vi "c ctre phoenixpro Request Control Position Voltage.vi"(0 "canbus":string, 1 "Position":dbl, 2 "FeedForward":dbl, 5 "ecuEncoding":u32, 7 "updateTime":dbl, 9 "cancelOtherRequests":bool, 11 "error in (no error)":errorcluster, 12 "EnableFOC":bool, 13 "Slot":i32) -> (4 "function return":i32, 15 "error out":errorcluster)   [LabVIEW 2020, in "CTRE_PhoenixTools.lvlib"]
doc: "CTREXPORT int c_ctre_phoenixpro_RequestControlPositionVoltage(const char *canbus, uint32_t ecuEncoding, double updateTime, bool cancelOtherRequests, double Position, bool EnableFOC, double FeedForward, int Slot);"
uses:
  <userlib>/CTRE_PhoenixTools/CTRE_PhoenixTools.lvlib
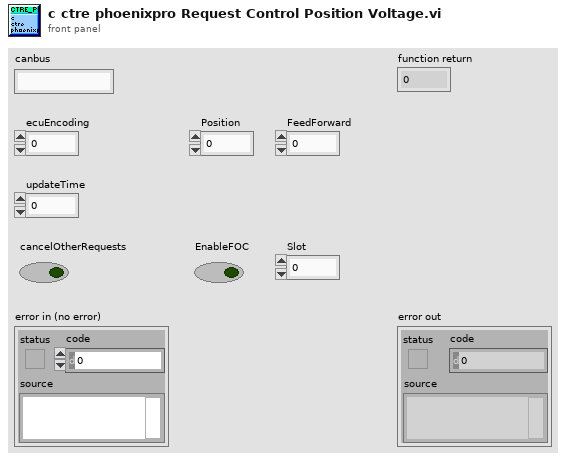
[diagram p1: front panel]
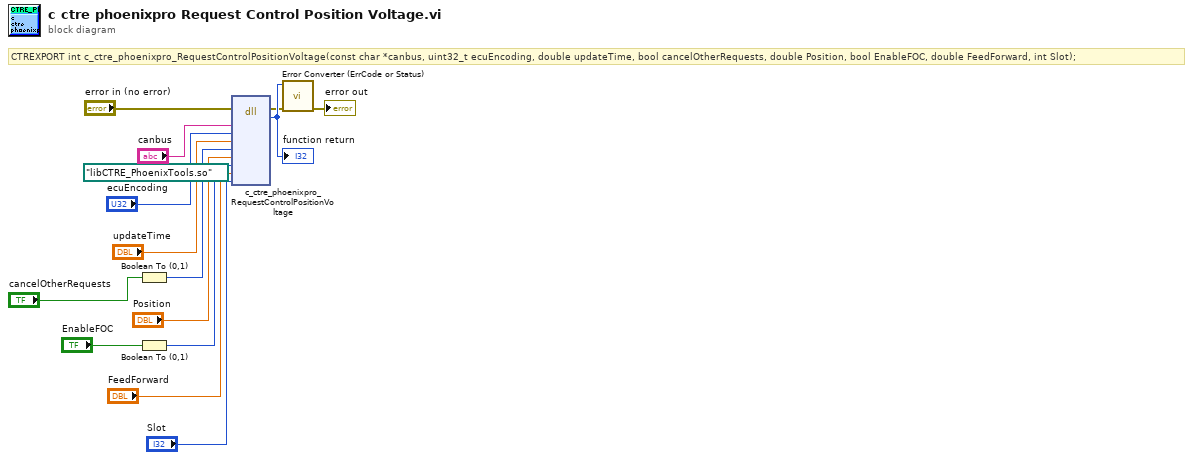
[diagram p0: block diagram]
diagram:
  # "CTREXPORT int c_ctre_phoenixpro_RequestControlPositionVoltage(const char *canbus, uint32_t ecuEncoding, double updateTime, bool cancelOtherRequests, double Position, bool EnableFOC, double FeedForward, int Slot);"
  n1 = Boolean To (0,1)(Boolean="cancelOtherRequests") -> (0, 1=w10:i16)
  n2 = Boolean To (0,1)(Boolean="EnableFOC") -> (0, 1=w7:i16)
  n3 = dll-call lib="?" fn="c_ctre_phoenixpro_RequestControlPositionVoltage"(path in=path "libCTRE_PhoenixTools.so", error in="error in (no error)", "canbus"="canbus", "ecuEncoding"="ecuEncoding", "updateTime"="updateTime", "cancelOtherRequests"=w10, "Position"="Position", "EnableFOC"=w7, "FeedForward"="FeedForward", "Slot"="Slot") -> (error out=w3:errorcluster, w15:i32)  [unwired: 9 in, 1 out]
  "function return" <- w15
  n4 = call <userlib>:"Error Converter (ErrCode or Status).vi"("error in (no error)"=w3, "error code"=w15) -> ("error out"=→"error out":errorcluster)  [unwired: 9 in]
